vi "FILTRO_FIR_MONO_V1.vi"() -> ()   [LabVIEW 2013]
uses:
  <vilib>/Analysis/3filter.llb/Filter Passband Type.ctl
  <vilib>/Analysis/4window.llb/windowTd.ctl
  <vilib>/Analysis/2dsp.llb/1D Convolution (DBL).vi
  <vilib>/Analysis/2dsp.llb/Real FFT.vi
  <vilib>/Analysis/NI_AALBase.lvlib
  <vilib>/Analysis/NI_AALPro.lvlib
panel:
  in  "FFT size":i32=512
  in  "shift?":bool=TRUE
  out "AUDIO_FILTRADO 2":dbl[](graph)=[0.15642497923002807, 0.15642973125237586, 0.1564296077155255, 0.15644363868987607, 0.15649654450679862, 0.15650889563989864, 0.1565262065198838, 0.15657242532025914, 0.15662047404122653, 0.1566675306236652, 0.15672018146199052, 0.15677661306772125, 0.15686256555785255, 0.15693329370988038, 0.1570124543705419, 0.15708831905725593, 0.1571888330114431, 0.15729747917147993, 0.15738826047087773, 0.15749443447761358, 0.15762012146635895, 0.15774034392520928, 0.1578778327697925, 0.15799626109587714, 0.15814398995770423, 0.15830552767769054, 0.15844836079196886, 0.15860970591352197, 0.1587736060356467, 0.15896044022992104, 0.1591373292068727, 0.15931827231675605, 0.15950049187994764, 0.15970835601934344, 0.15992615789489642, 0.16012295677372237, 0.16033582200998897, 0.1605713913205365, 0.16080904520103656, 0.16104503734917508, 0.16128014130632615, 0.1615340401398511, 0.16181502363544206, 0.16207502524231612, 0.16233491761364885, 0.16261600505390464, 0.16292314635297564, 0.16320764826798306, 0.1635053641895551, 0.1638108710762677, 0.1641365396427896, 0.16445779818300674, 0.16479517571539004, 0.16512635457396221, 0.16548515936530273, 0.16584521013499745, 0.16619710357744208, 0.16656089280633937, 0.1669522731184149, 0.16734790691805873, 0.16773958629725574, 0.16812682135386875, 0.1685313688619773, 0.16896366923257852, 0.1694280073096003, 0.16983363753803418, 0.17028185798315573, 0.1707469435180873, 0.17122294541955185, 0.17167975094788468, 0.17215377002281507, 0.172668656829585, 0.17316858978899594, 0.1737022546210849, 0.17418337405165288, 0.17474303254254117, 0.1753377845468974, 0.1758471599361695, 0.17637035657473965, 0.17696579865105702, 0.17752102181661553, 0.17811047753413514, 0.17870150980726607, 0.17930896903282106, 0.17995592284775042, 0.18065434398758018, 0.18122982421858627, 0.1818760821910609, 0.18261225777327447, 0.18325479920695864, 0.1839348115431484, 0.18467551624887557, 0.18532719424129876, 0.18611506753032667, 0.18686638362466762, 0.1875897586488568, 0.18836185512894774, 0.18918473830382154, 0.18997425484119324, 0.19076817492729936, 0.19159332862551906, 0.1925458411586536, 0.19327909563255583, 0.19418277340400336, 0.19502055626555326, 0.19600229084028817, 0.19694419444404088, 0.19784990808634895, 0.1988010605938312, 0.1997854468638729, 0.20067678671589775, 0.20176490573771055, 0.20278646911199152, 0.20378581063033788, 0.20484278066226222, 0.20590553937698916, 0.20698284182627702, 0.20813371946516512, 0.20929854741605947, 0.21053769206733458, 0.2116455059677825, 0.2129825297072197, 0.21406345269321983, 0.2153636078527049, 0.21661585438086026, 0.21776161752819348, 0.2191994261784744, 0.22054801187151618, 0.22190363494125925, 0.22331542178048688, 0.22471979699478772, 0.22620604484412132, 0.2276256427082507, 0.22912448292679977, 0.23058601140391552, 0.23229858435271764, 0.23395718681817737, 0.23548721135935433, 0.2370381741296052, 0.23885557546255753, 0.24063588509550052, 0.24226877231999394, 0.2441793400393237, 0.24616099999294683, 0.24781068082045907, 0.2497519988307107, 0.2516079111341652, 0.2537396251762966, 0.2558106464751237, 0.2578546039944259, 0.2598700288914405, 0.26217418760802125, 0.2643629755631493, 0.2666271577768467, 0.26880748903367363, 0.2714832991443721, 0.2735720452381094, 0.2762103778161411, 0.2785884779525825, 0.2814362309427154, 0.2841201412978474, 0.28659347819511954, 0.28948303621371185, 0.29221246065334455, 0.2960707804491421, 0.2982640501004512, 0.3013459631528612, 0.30457946689430554, 0.30790261423014237, 0.3110109304486261, 0.3146995027209519, 0.31864707285666294, 0.32173248260223236, 0.32556207173657536, 0.3297717039403118, 0.3332641985740337, 0.337777524158535, 0.34183754879131206, 0.34653404957457784, 0.35104607263603854, 0.35543800720582036, 0.36061453476826943, 0.3659263343213047, 0.37210262144986317, 0.377603534520562, 0.38339606180295605, 0.39020357154712976, 0.39753735415629876, 0.4041250373561819, 0.40633896703832534, 0.43680860160990115, 0.47880835666900956, 0.48452781371836734, 0.37917850639793327, 0.32778865022285897, 0.8494102555902882, 0.2608733554574993, 0.42069254617843, 0.9340591257737484, 0.8489546266948398, 0.8573284294543184, 0.8187114491191063, 0.4139708431755166, 0.8238776676961604, 1.232811763327611, 1.7342419461026934, 0.9494714908595501, 1.3322682388273699, 1.4846538528126787, 1.503003911075233, 1.3458292982137192, 1.0018998576392086, 2.306406615040041, 1.1048144820955037, 1.198955434392726, 2.9064288725794176, 1.9036619986351853, 1.3999755190121836, 2.3245725979848846, 0.40914527294823505, 0.11689024378423747, 0.9929579036437363, 1.4056263369388868, 0.17094077172810287, 0.5310250932149697, 4.413554363722428, 1.938227684647852, 1.728884107646817, 1.3387636871837514, 0.7603278801346938, 1.307661788954466, 1.8438949954431731, 1.4683818778407476, 4.566324440230887, 3.0163273704827795, 3.864243886270696, 1.4760886810436533, 2.034510092951714, 3.1403320629455473, 1.3176218140270874, 1.5142069537579288, 3.0096019895042208, 1.7530761962052754, 3.5050023570559508, 6.890058644447735, 1.063761809719905, 8.255401404916554, 5.436012977595252, 4.958923738284641, 7.1928532757213155, 13.259982742156541, 10.338683128858044, 23.44413146941271, 36.093188344927334, 46.36519505994677, 91.37086850984034, 38.7867849922724, 91.37086850984034, 46.36519505994677, 36.093188344927334, 23.44413146941271, 10.338683128858044, 13.259982742156541, 7.1928532757213155, 4.958923738284641, 5.436012977595252, 8.255401404916554, 1.063761809719905, 6.890058644447735, 3.5050023570559508, 1.7530761962052754, 3.0096019895042208, 1.5142069537579288, 1.3176218140270874, 3.1403320629455473, 2.034510092951714, 1.4760886810436533, 3.864243886270696, 3.0163273704827795, 4.566324440230887, 1.4683818778407476, 1.8438949954431731, 1.307661788954466, 0.7603278801346938, 1.3387636871837514, 1.728884107646817, 1.938227684647852, 4.413554363722428, 0.5310250932149697, 0.17094077172810287, 1.4056263369388868, 0.9929579036437363, 0.11689024378423747, 0.40914527294823505, 2.3245725979848846, 1.3999755190121836, 1.9036619986351853, 2.9064288725794176, 1.198955434392726, 1.1048144820955037, 2.306406615040041, 1.0018998576392086, 1.3458292982137192, 1.503003911075233, 1.4846538528126787, 1.3322682388273699, 0.9494714908595501, 1.7342419461026934, 1.232811763327611, 0.8238776676961604, 0.4139708431755166, 0.8187114491191063, 0.8573284294543184, 0.8489546266948398, 0.9340591257737484, 0.42069254617843, 0.2608733554574993, 0.8494102555902882, 0.32778865022285897, 0.37917850639793327, 0.48452781371836734, 0.47880835666900956, 0.43680860160990115, 0.40633896703832534, 0.4041250373561819, 0.39753735415629876, 0.39020357154712976, 0.38339606180295605, 0.377603534520562, 0.37210262144986317, 0.3659263343213047, 0.36061453476826943, 0.35543800720582036, 0.35104607263603854, 0.34653404957457784, 0.34183754879131206, 0.337777524158535, 0.3332641985740337, 0.3297717039403118, 0.32556207173657536, 0.32173248260223236, 0.31864707285666294, 0.3146995027209519, 0.3110109304486261, 0.30790261423014237, 0.30457946689430554, 0.3013459631528612, 0.2982640501004512, 0.2960707804491421, 0.29221246065334455, 0.28948303621371185, 0.28659347819511954, 0.2841201412978474, 0.2814362309427154, 0.2785884779525825, 0.2762103778161411, 0.2735720452381094, 0.2714832991443721, 0.26880748903367363, 0.2666271577768467, 0.2643629755631493, 0.26217418760802125, 0.2598700288914405, 0.2578546039944259, 0.2558106464751237, 0.2537396251762966, 0.2516079111341652, 0.2497519988307107, 0.24781068082045907, 0.24616099999294683, 0.2441793400393237, 0.24226877231999394, 0.24063588509550052, 0.23885557546255753, 0.2370381741296052, 0.23548721135935433, 0.23395718681817737, 0.23229858435271764, 0.23058601140391552, 0.22912448292679977, 0.2276256427082507, 0.22620604484412132, 0.22471979699478772, 0.22331542178048688, 0.22190363494125925, 0.22054801187151618, 0.2191994261784744, 0.21776161752819348, 0.21661585438086026, 0.2153636078527049, 0.21406345269321983, 0.2129825297072197, 0.2116455059677825, 0.21053769206733458, 0.20929854741605947, 0.20813371946516512, 0.20698284182627702, 0.20590553937698916, 0.20484278066226222, 0.20378581063033788, 0.20278646911199152, 0.20176490573771055, 0.20067678671589775, 0.1997854468638729, 0.1988010605938312, 0.19784990808634895, 0.19694419444404088, 0.19600229084028817, 0.19502055626555326, 0.19418277340400336, 0.19327909563255583, 0.1925458411586536, 0.19159332862551906, 0.19076817492729936, 0.18997425484119324, 0.18918473830382154, 0.18836185512894774, 0.1875897586488568, 0.18686638362466762, 0.18611506753032667, 0.18532719424129876, 0.18467551624887557, 0.1839348115431484, 0.18325479920695864, 0.18261225777327447, 0.1818760821910609, 0.18122982421858627, 0.18065434398758018, 0.17995592284775042, 0.17930896903282106, 0.17870150980726607, 0.17811047753413514, 0.17752102181661553, 0.17696579865105702, 0.17637035657473965, 0.1758471599361695, 0.1753377845468974, 0.17474303254254117, 0.17418337405165288, 0.1737022546210849, 0.17316858978899594, 0.172668656829585, 0.17215377002281507, 0.17167975094788468, 0.17122294541955185, 0.1707469435180873, 0.17028185798315573, 0.16983363753803418, 0.1694280073096003, 0.16896366923257852, 0.1685313688619773, 0.16812682135386875, 0.16773958629725574, 0.16734790691805873, 0.1669522731184149, 0.16656089280633937, 0.16619710357744208, 0.16584521013499745, 0.16548515936530273, 0.16512635457396221, 0.16479517571539004, 0.16445779818300674, 0.1641365396427896, 0.1638108710762677, 0.1635053641895551, 0.16320764826798306, 0.16292314635297564, 0.16261600505390464, 0.16233491761364885, 0.16207502524231612, 0.16181502363544206, 0.1615340401398511, 0.16128014130632615, 0.16104503734917508, 0.16080904520103656, 0.1605713913205365, 0.16033582200998897, 0.16012295677372237, 0.15992615789489642, 0.15970835601934344, 0.15950049187994764, 0.15931827231675605, 0.1591373292068727, 0.15896044022992104, 0.1587736060356467, 0.15860970591352197, 0.15844836079196886, 0.15830552767769054, 0.15814398995770423, 0.15799626109587714, 0.1578778327697925, 0.15774034392520928, 0.15762012146635895, 0.15749443447761358, 0.15738826047087773, 0.15729747917147993, 0.1571888330114431, 0.15708831905725593, 0.1570124543705419, 0.15693329370988038, 0.15686256555785255, 0.15677661306772125, 0.15672018146199052, 0.1566675306236652, 0.15662047404122653, 0.15657242532025914, 0.1565262065198838, 0.15650889563989864, 0.15649654450679862, 0.15644363868987607, 0.1564296077155255, 0.15642973125237586]
  out "AUDIO_SIN_FILTRAR":waveform(dbl)(graph)={"t0"=timestamp(3508764430.541633 s since 1904-01-01), "dt"=2.266999999999997e-05, "Y"=array[44104 elements], "attributes"=variant("NI_ChannelName"=variant(string "Voltage"), "NI_UnitDescription"=variant(string "Volts"))}
  out "AUDIO_FILTRADO":waveform(dbl)(graph)={"t0"=timestamp(3508764430.541633 s since 1904-01-01), "dt"=2.266999999999997e-05, "Y"=array[44224 elements]}
  out "FIR Windowed Coefficients":dbl[](array[numeric])=[-0.00019115936790040078, -0.00027601762453655613, -0.00022538960724483769, -3.274865467090994e-05, 0.00022831832692832223, 0.00042600379398731355, 0.00043149349904345746, 0.00019383727718514534, -0.00021154977061043574, -0.0005952944005058377, -0.0007349542546577839, -0.0004941189129628715, 7.9772032249903e-05, 0.0007399675383366554, 0.0011350116392557915, 0.0009842117076873619, 0.00025191629005409715, -0.0007788372254998085, -0.0015969362698426885, -0.0017018260827114798, -0.0008864114913413695, 0.0005862353461644945, 0.0020336935471596423, 0.0026500698524301704, 0.0019299669776700202, 8.497153848166417e-06, -0.0022889719968409426, -0.0037709672393248512, -0.003468762728042707, -0.0012128126374511283, 0.002124874683274546, 0.004917853294223526, 0.0055398895001038855, 0.003256137956731042, -0.0012140824825521348, -0.005829386201973178, -0.00810332645957702, -0.006378457931204458, -0.0008738877475532727, 0.0061006704316331865, 0.011023690527389314, 0.01084815612889383, 0.004729253757509455, -0.005122915936124375, -0.014070219351340523, -0.017077218427437372, -0.011321441339295388, 0.0018791017076534831, 0.01693993907228761, 0.026069838030011103, 0.022863755385628907, 0.005915393486017005, -0.019302778942971336, -0.04146816136109546, -0.0473151239037303, -0.02705990255150618, 0.020860315540480824, 0.08785994102835461, 0.15718009888382767, 0.20926786867165365, 0.22859561028712563, 0.20926786867165365, 0.15718009888382767, 0.08785994102835461, 0.020860315540480824, -0.02705990255150618, -0.0473151239037303, -0.04146816136109546, -0.019302778942971336, 0.005915393486017005, 0.022863755385628907, 0.026069838030011103, 0.01693993907228761, 0.0018791017076534831, -0.011321441339295388, -0.017077218427437372, -0.014070219351340523, -0.005122915936124375, 0.004729253757509455, 0.01084815612889383, 0.011023690527389314, 0.0061006704316331865, -0.0008738877475532727, -0.006378457931204458, -0.00810332645957702, -0.005829386201973178, -0.0012140824825521348, 0.003256137956731042, 0.0055398895001038855, 0.004917853294223526, 0.002124874683274546, -0.0012128126374511283, -0.003468762728042707, -0.0037709672393248512, -0.0022889719968409426, 8.497153848166417e-06, 0.0019299669776700202, 0.0026500698524301704, 0.0020336935471596423, 0.0005862353461644945, -0.0008864114913413695, -0.0017018260827114798, -0.0015969362698426885, -0.0007788372254998085, 0.00025191629005409715, 0.0009842117076873619, 0.0011350116392557915, 0.0007399675383366554, 7.9772032249903e-05, -0.0004941189129628715, -0.0007349542546577839, -0.0005952944005058377, -0.00021154977061043574, 0.00019383727718514534, 0.00043149349904345746, 0.00042600379398731355, 0.00022831832692832223, -3.274865467090994e-05, -0.00022538960724483769, -0.00027601762453655613, -0.00019115936790040078]
  in  "number of samples":i32=44104
  in  "rate":dbl=44100.0
  out "error":i32
  in  "FRECUENCIA\nDE CORTE\nINFERIOR":dbl(slide)=5040.53320683112 scale=1.0..16000.0
  in  "FRECUENCIA\nDE CORTE\nSUPERIOR":dbl(slide)=1184.9867172675522 scale=1.0..16000.0
  in  "window parameter":dbl=nan
  in  "option":enum32{"not scaled", "scaled"}(ring)
  in  "window":T1=62 items=["Rectangle"=0, "Hanning"=1, "Hamming"=2, "Blackman-Harris"=3, "Exact Blackman"=4, "Blackman"=5, "Flat Top"=6, "4 Term B-Harris "=7, "7 Term B-Harris"=8, "Low Sidelobe"=9, "Blackman Nuttall"=11, "Triangle"=30, "Bartlett-Hanning"=31, "Bohman"=32, "Parzen"=33, "Welch"=34, "Kaiser"=60, "Dolph-Chebyshev"=61, "Gaussian"=62]
  in  "taps":i32=121 min=1
  in  "sampling freq: fs":dbl=44100.0 format="%0.2f"
  in  "filter type":T2
  out "?":string="FILTRADO"
  in  "¿FILTRADO?":bool=TRUE
  out "error out":errorcluster
  in  "stop":bool
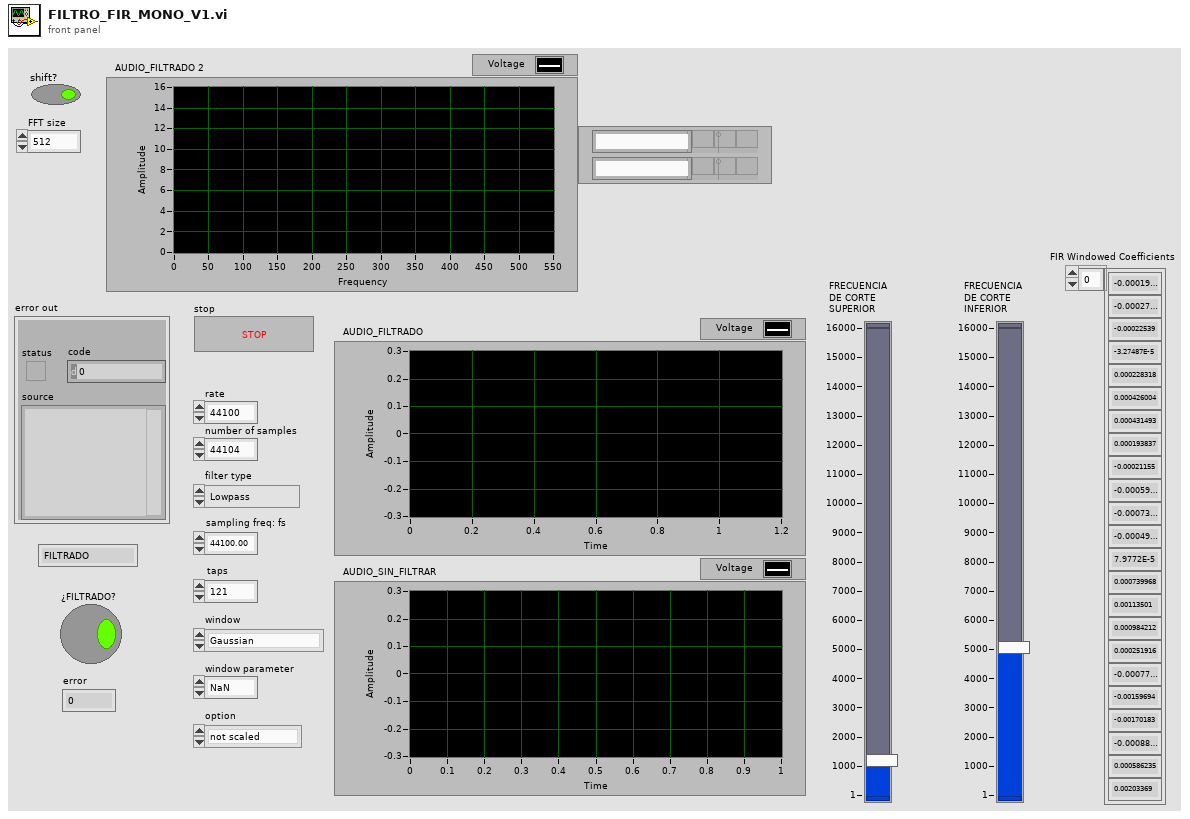
[diagram p1: front panel]
types:
  T1 = typedef "NI_AALPro.lvlib/windowTd.ctl" = u32
  T2 = typedef "NI_AALBase.lvlib/Filter Passband Type.ctl" = enum32{"Lowpass", "Highpass", "Bandpass", "Bandstop"}
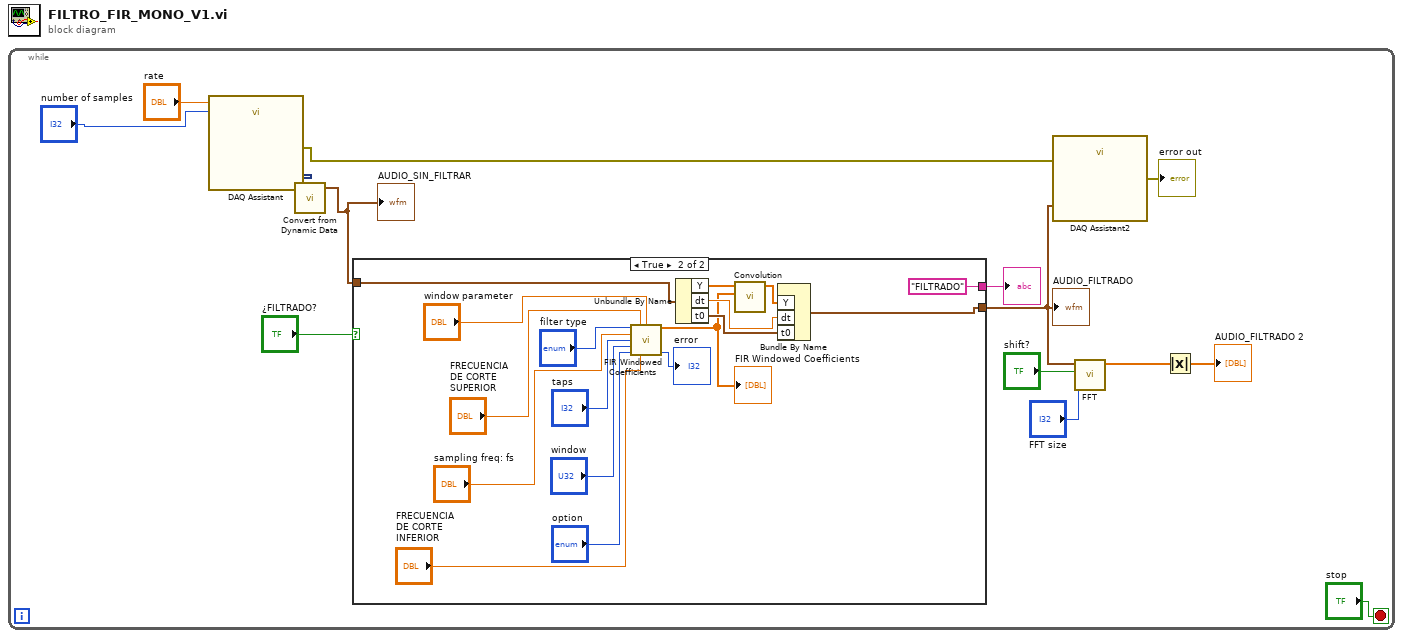
[diagram p0: block diagram]
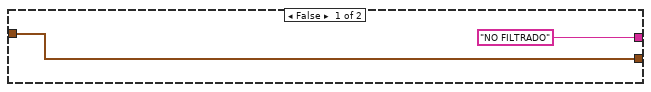
[diagram p2: hidden frame]
diagram:
  n1 = while {
    stop <- "stop" stop-if-true
    n2 = call "DAQ Assistant"("rate"="rate", "number of samples"="number of samples") -> ("data"=w11:dynamicdata, "error out"=w13:errorcluster)  [unwired: 14 in, 2 out]
    n3 = call "Convert from Dynamic Data"("Dynamic Data Type"=w11) -> ("Waveform"=w6:waveform(dbl))  [unwired: 3 in]
    "AUDIO_SIN_FILTRAR" <- w6
    n4 = case shown="True" "¿FILTRADO?" {
      tunnel: ["NO FILTRADO" "FILTRADO"] -> w9
      tunnel: w6 -> [w15 w26]
      tunnel: [w15 w23] -> w5
      frame False {
      }
      frame True {
        n5 = call <vilib>:"FIR Windowed Coefficients.vi"("filter type"="filter type", "high cutoff freq: fh"="FRECUENCIA\nDE CORTE\nSUPERIOR", "window parameter"="window parameter", "sampling freq: fs"="sampling freq: fs", "taps"="taps", "window"="window", "option"="option", "low cutoff freq: fl"="FRECUENCIA\nDE CORTE\nINFERIOR") -> ("FIR Windowed Coefficients"=w21:dbl[], "error"=→"error":i32)  [unwired: 6 in]
        "FIR Windowed Coefficients" <- w21
        n6 = Unbundle By Name(w26) -> ("Y"=w22:dbl[], "dt"=w25:dbl, "t0"=w24:timestamp)
        n7 = call-poly <vilib>:"Convolution.vi"("Y"=w21, "X"=w22) -> ("X * Y"=w20:dbl[])  [unwired: 8 in, 1 out]
        n8 = Bundle By Name("Y"=w20, "dt"=w25, "t0"=w24) -> (w23:waveform(dbl))  [unwired: 1 in]
      }
    }
    "?" <- w9
    "AUDIO_FILTRADO" <- w5
    n9 = call "DAQ Assistant2"("data"=w5, "error in"=w13) -> ("error out"=→"error out":errorcluster)  [unwired: 15 in, 2 out]
    n10 = call-poly <vilib>:"FFT.vi"("FFT size"="FFT size", "shift?"="shift?", "X"=w5) -> ("FFT {X}"=w4:cdb[])  [unwired: 7 in, 1 out]
    n11 = Absolute Value(x=w4) -> (abs(x)=→"AUDIO_FILTRADO 2":dbl[])
  }
